vi "range_to_number_sub.vi"(11 "Characters Read":string) -> (3 "Numeric":i32)   [LabVIEW 2021]
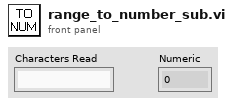
[diagram p1: front panel]
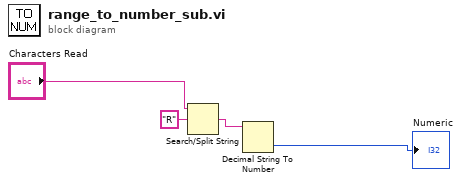
[diagram p0: block diagram]
diagram:
  n1 = Search/Split String(string="Characters Read", search string/char (-)="R") -> (match + rest of string=w2:string)  [unwired: 1 in, 2 out]
  n2 = Decimal String To Number(string=w2) -> (number=→"Numeric":i32)  [unwired: 2 in, 1 out]
